vi "LB_NameArray.vi"(11 "error in (no error)":errorcluster) -> (15 "error out":errorcluster)   [LabVIEW 2016, in "DronaTest.lvlib"]
uses:
  DronaTest.lvlib
  APIs/Stimulus/ControlValue/Controls/Listbox/typedef/Name&Occuuence.ctl
  APIs/Stimulus/ControlValue/SetValueAuto.vi
  APIs/Stimulus/ControlValue/Controls/Listbox/SetValueByArrayName.vi
  APIs/Assert/AssertControlValue/Equal.vi
  <vilib>/addons/_JKI Toolkits/Caraya/classes/Assert/Assert Error.vi
  APIs/Stimulus/VI/CloseVI.vi
  <vilib>/addons/_JKI Toolkits/Caraya/classes/Test/Test.lvclass
  Drona.lvlib
  <vilib>/SLL Toolkit/SLL Debug/SLL Debug.lvlib
  APIs/Stimulus/ControlValue/Controls/Listbox/StimulusListbox.lvlib
  APIs/Stimulus/ControlValue/ControlValue.lvlib
  APIs/Assert/AssertControlValue/AssertControlValue.lvlib
  <vilib>/addons/_JKI Toolkits/Caraya/classes/Assert/Assert.lvclass
  APIs/Stimulus/VI/VI.lvlib
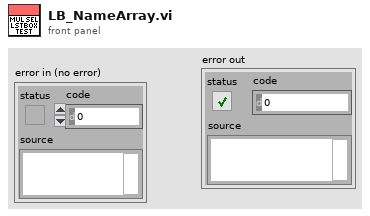
[diagram p1: front panel]
types:
  T1 = typedef "Drona.lvlib/ControlValue.lvlib/StimulusListbox.lvlib/Name&Occuuence.ctl" = cluster{"ItemName":string, "Occurrence":i32}
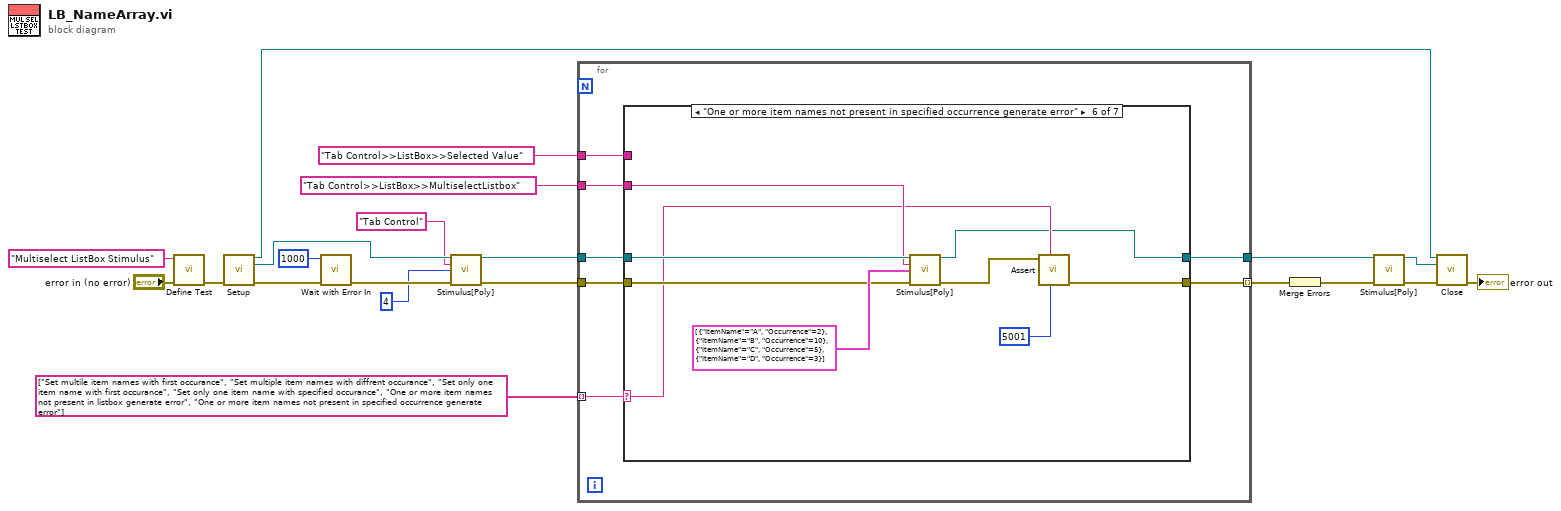
[diagram p0: block diagram]
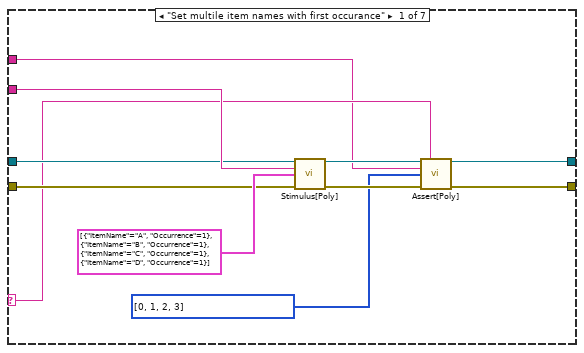
[diagram p2: hidden frame]
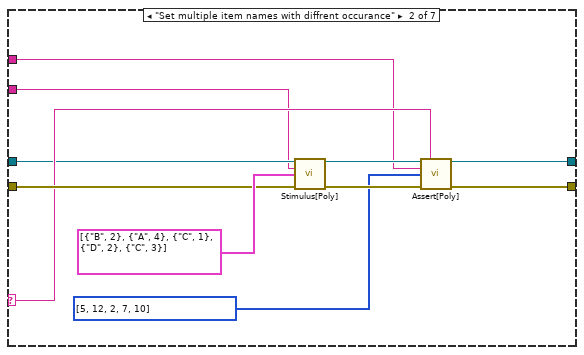
[diagram p3: hidden frame]
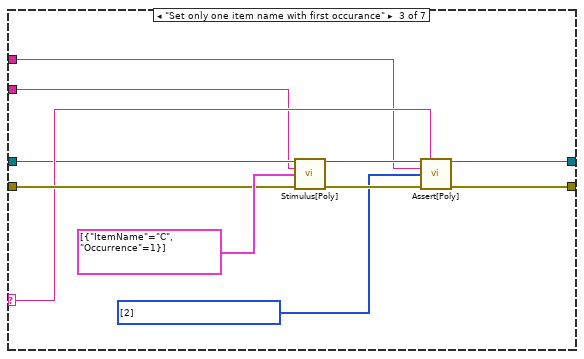
[diagram p4: hidden frame]
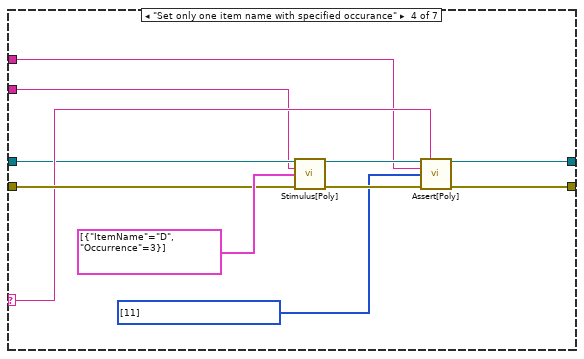
[diagram p5: hidden frame]
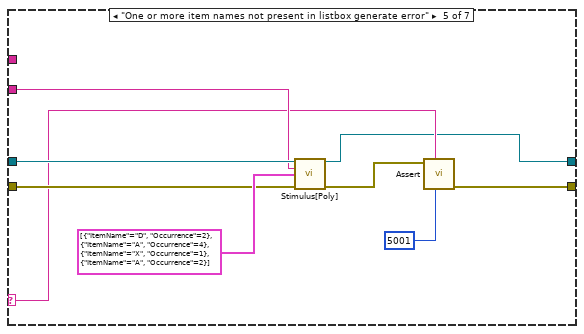
[diagram p6: hidden frame]
diagram:
  n1 = call <vilib>:"Define Test.vi"("error in (no error)"="error in (no error)", "Label (VI Title)"="Multiselect ListBox Stimulus") -> ("error out"=w20:errorcluster)  [unwired: 9 in]
  n2 = call "Setup.vi"("error in"=w20) -> ("Application Ref"=w5:refnum<vi>, "VI Reference Out"=w15:refnum<vi>, "error out"=w19:errorcluster)  [unwired: 12 in]
  n3 = call <vilib>:"Wait with Error In.vi"("error in (no error)"=w19, "milliseconds to wait"=u32 1000) -> ("error out"=w16:errorcluster)  [unwired: 9 in]
  n4 = call-poly "Stimulus[Poly].vi"("VI Reference In"=w15, "Control Path"="Tab Control", "Value (Signaling)"=4, "error in"=w16) -> ("VI Reference Out"=w7:refnum<vi>, "error out"=w6:errorcluster)  [unwired: 10 in]
  n5 = for {
    tunnel: [w28] -> w4 mode=indexing
    tunnel: [w27] -> w9
    tunnel: string[] ["Set multile item names with first occurance", "Set multiple item names with diffrent occurance", "Set only one item name with first occurance", "Set only one item name with specified occurance", "One or more item names not present in listbox generate error", "One or more item names not present in specified occurrence generate error"] -> [w26] mode=indexing
    tunnel: w7 -> [w25]
    tunnel: w6 -> [w24]
    tunnel: "Tab Control>>ListBox>>MultiselectListbox" ("Control Path") -> [w23]
    tunnel: "Tab Control>>ListBox>>Selected Value" ("Control Path") -> [w22]
    n6 = case shown="\"One or more item names not present in specified occurrence generate error\"" w26 {
      selector: w26 -> [w30 w43 w54 w65 w74 w83 _]
      tunnel: [w39 w50 w61 w72 w76 w85 w91] -> w28
      tunnel: [w38 w49 w60 w71 w73 w82 w92] -> w27
      tunnel: w25 -> [w31 w42 w53 w64 w79 w88 w92]
      tunnel: w24 -> [w33 w44 w55 w66 w80 w89 w91]
      tunnel: w23 -> [w32 w41 w52 w63 w78 w87 _]
      tunnel: w22 -> [w29 w40 w51 w62 _ _ _]
      frame "Set multile item names with first occurance" {
        n7 = call-poly "Stimulus[Poly].vi"("VI Reference In"=w31, "Control Path"=w32, "Name Array"=T1[] [{"ItemName"="A", "Occurrence"=1}, {"ItemName"="B", "Occurrence"=1}, {"ItemName"="C", "Occurrence"=1}, {"ItemName"="D", "Occurrence"=1}], "Error In"=w33) -> ("VI Reference Out"=w36:refnum<vi>, "Error Out"=w37:errorcluster)  [unwired: 10 in]
        n8 = call-poly "Assert[Poly].vi"("VI Reference In"=w36, "Test Label"=w30, "Control Path"=w29, "Control Value"=i32[] [0, 1, 2, 3] ("Index Array"), "Error In"=w37) -> ("VI Reference Out"=w38:refnum<vi>, "Error Out"=w39:errorcluster)  [unwired: 8 in, 1 out]
      }
      frame "Set multiple item names with diffrent occurance" {
        n9 = call-poly "Stimulus[Poly].vi"("VI Reference In"=w42, "Control Path"=w41, "Name Array"=T1[] [{"ItemName"="B", "Occurrence"=2}, {"ItemName"="A", "Occurrence"=4}, {"ItemName"="C", "Occurrence"=1}, {"ItemName"="D", "Occurrence"=2}, {"ItemName"="C", "Occurrence"=3}], "Error In"=w44) -> ("VI Reference Out"=w47:refnum<vi>, "Error Out"=w48:errorcluster)  [unwired: 10 in]
        n10 = call-poly "Assert[Poly].vi"("VI Reference In"=w47, "Test Label"=w43, "Control Path"=w40, "Control Value"=i32[] [5, 12, 2, 7, 10] ("Index Array"), "Error In"=w48) -> ("VI Reference Out"=w49:refnum<vi>, "Error Out"=w50:errorcluster)  [unwired: 8 in, 1 out]
      }
      frame "Set only one item name with first occurance" {
        n11 = call-poly "Stimulus[Poly].vi"("VI Reference In"=w53, "Control Path"=w52, "Name Array"=T1[] [{"ItemName"="C", "Occurrence"=1}], "Error In"=w55) -> ("VI Reference Out"=w58:refnum<vi>, "Error Out"=w59:errorcluster)  [unwired: 10 in]
        n12 = call-poly "Assert[Poly].vi"("VI Reference In"=w58, "Test Label"=w54, "Control Path"=w51, "Control Value"=i32[] [2] ("Index Array"), "Error In"=w59) -> ("VI Reference Out"=w60:refnum<vi>, "Error Out"=w61:errorcluster)  [unwired: 8 in, 1 out]
      }
      frame "Set only one item name with specified occurance" {
        n13 = call-poly "Stimulus[Poly].vi"("VI Reference In"=w64, "Control Path"=w63, "Name Array"=T1[] [{"ItemName"="D", "Occurrence"=3}], "Error In"=w66) -> ("VI Reference Out"=w69:refnum<vi>, "Error Out"=w70:errorcluster)  [unwired: 10 in]
        n14 = call-poly "Assert[Poly].vi"("VI Reference In"=w69, "Test Label"=w65, "Control Path"=w62, "Control Value"=i32[] [11] ("Index Array"), "Error In"=w70) -> ("VI Reference Out"=w71:refnum<vi>, "Error Out"=w72:errorcluster)  [unwired: 8 in, 1 out]
      }
      frame "One or more item names not present in listbox generate error" {
        n15 = call-poly "Stimulus[Poly].vi"("VI Reference In"=w79, "Control Path"=w78, "Name Array"=T1[] [{"ItemName"="D", "Occurrence"=2}, {"ItemName"="A", "Occurrence"=4}, {"ItemName"="X", "Occurrence"=1}, {"ItemName"="A", "Occurrence"=2}], "Error In"=w80) -> ("VI Reference Out"=w73:refnum<vi>, "Error Out"=w77:errorcluster)  [unwired: 10 in]
        n16 = call-poly <vilib>:"Assert.vi"("error code (1)"=5001, "Label"=w74, "Error?"=w77) -> ("error out"=w76:errorcluster)  [unwired: 8 in]
      }
      frame "One or more item names not present in specified occurrence generate error" {
        n17 = call-poly "Stimulus[Poly].vi"("VI Reference In"=w88, "Control Path"=w87, "Name Array"=T1[] [{"ItemName"="A", "Occurrence"=2}, {"ItemName"="B", "Occurrence"=10}, {"ItemName"="C", "Occurrence"=5}, {"ItemName"="D", "Occurrence"=3}], "Error In"=w89) -> ("VI Reference Out"=w82:refnum<vi>, "Error Out"=w86:errorcluster)  [unwired: 10 in]
        n18 = call-poly <vilib>:"Assert.vi"("error code (1)"=5001, "Label"=w83, "Error?"=w86) -> ("error out"=w85:errorcluster)  [unwired: 8 in]
      }
      frame Default {
      }
    }
  }
  n19 = Merge Errors(w4) -> (w3:errorcluster)
  n20 = call-poly "Stimulus[Poly].vi"("VI Reference In"=w9, "error in"=w3) -> ("VI Reference Out"=w11:refnum<vi>, "error out"=w10:errorcluster)  [unwired: 12 in]
  n21 = call "Close.vi"("Application Ref"=w5, "VI Reference"=w11, "error in"=w10) -> ("error out"=→"error out":errorcluster)  [unwired: 12 in]
